vi "MTMount_registerCallback_logEvent_axesInPosition.vi"(8 "error in (no error)":errorcluster, 10 "skipOld":bool, 11 "handle":i32) -> (0 "error out":errorcluster, 3 "function return":i32)   [LabVIEW 2018, in "SALLV_MTMount.lvlib"]
doc: "int MTMount_shm_registerCallback_logevent_axesInPositionLV(int handle, bool skipOld);"
uses:
  SALLV_MTMount.lvlib
  SALLV_MTMount.so
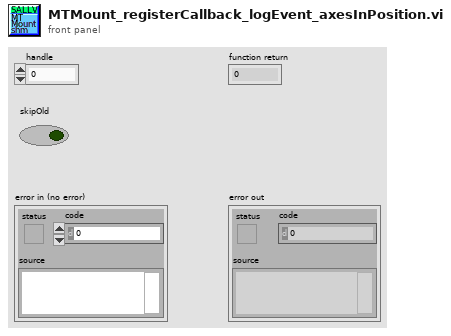
[diagram p1: front panel]
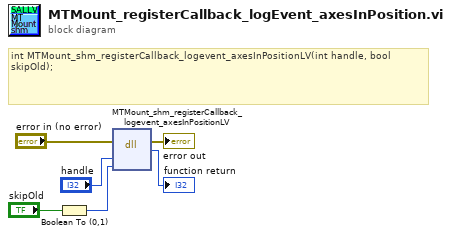
[diagram p0: block diagram]
diagram:
  # "int MTMount_shm_registerCallback_logevent_axesInPositionLV(int handle, bool skipOld);"
  n1 = Boolean To (0,1)(Boolean="skipOld") -> (0, 1=w3:i16)
  n2 = dll-call lib="home/ttsai/Documents/salLabviewApi/SALLV_MTMount/SALLV_MTMount.*" fn="MTMount_shm_registerCallback_logevent_axesInPositionLV"(error in="error in (no error)", "handle"="handle", "skipOld"=w3) -> (error out=→"error out":errorcluster, →"function return":i32)  [unwired: 4 in, 1 out]
